vi "DateTimeStringToTableName.vi"(2 "error in":errorcluster, 3 "Time String":string, 4 "Date String":string) -> (0 "error out":errorcluster, 1 "Table Name":string)   [LabVIEW 2023]
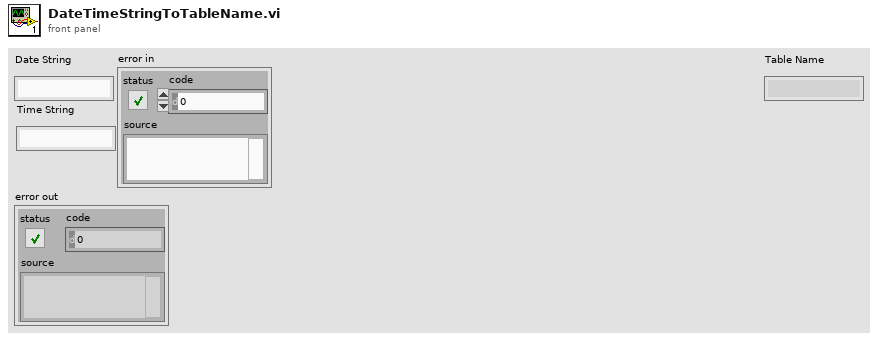
[diagram p1: front panel]
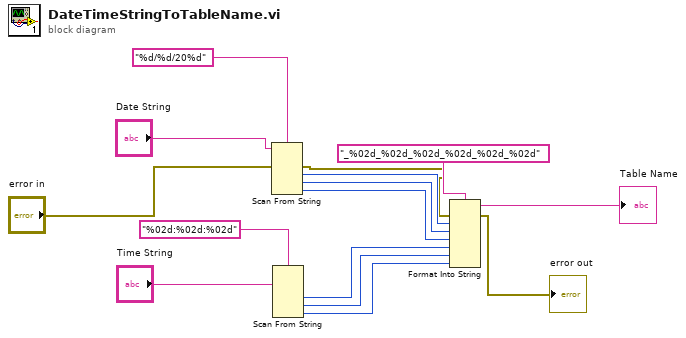
[diagram p0: block diagram]
diagram:
  n1 = Scan From String(format string="%d/%d/20%d", input string="Date String", error in="error in") -> (error out=w1:errorcluster, output 1=w10:i32, output 2=w9:i32, output 3=w8:i32)  [unwired: 4 in, 2 out]
  n2 = Scan From String(format string="%02d:%02d:%02d", input string="Time String") -> (output 1=w7:i32, output 2=w6:i32, output 3=w5:i32)  [unwired: 5 in, 3 out]
  n3 = Format Into String(format string="_%02d_%02d_%02d_%02d_%02d_%02d" ("time format string (%c)"), error in=w1, w10, w9, w8, w7, w6, w5) -> (resulting string=→"Table Name":string, error out=→"error out":errorcluster)  [unwired: 1 in]
